vi "PCAN_WRITE.vi"(7 "path in":path, 8 "error in (no error)":errorcluster, 11 "TPCANMsg":T1={"ID"=0, "MSGTYPE"=128, "LEN"=0, "Data"=[]} {"ID" format="%x"; "MSGTYPE" items=["STATUS"=128, "EXTENDED"=2, "RTR"=1, "DATA MSG"=0]}) -> (0 "error out":errorcluster, 2 "path out":path, 3 "error":T2 items=["CAN_ERR_OK"=0, "CAN_ERR_XMTFULL"=1, "CAN_ERR_OVERRUN"=2, "CAN_ERR_BUSLIGHT"=4, "CAN_ERR_BUSHEAVY"=8, "CAN_ERR_BUSOFF"=16, "CAN_ERR_QRCVEMPTY"=32, "CAN_ERR_QOVERRUN"=64, "CAN_ERR_QXMTFULL"=128, "CAN_ERR_REGTEST"=256, "CAN_ERR_NOVXD"=512, "CAN_ERR_HWINUSE"=1024, "CAN_ERR_NETINUSE"=2048, "CAN_ERR_ILLHW"=5120, "CAN_ERR_ILLNET"=6144, "CAN_ERR_ILLCLINET"=7168, "CAN_ERR_RESOURCE"=8192, "CAN_ERR_ILLPARAMTYPE"=16384, "CAN_ERR_ILLPARAMVAL"=32768, "CAN_ERR_UNKNOWN"=65536])   [LabVIEW 2017]
doc: "///////////////////////////////////////////////////////////////////////////////\n// CAN_Write()\n// Schreibt eine Message \n// moegliche Fehler: NOVXD RESOURCE BUSOFF QXMTFULL\n//\n\nDWORD __stdcall CAN_Write( TPCANMsg* pMsgBuff);"
uses:
  PCAN_ERROR.ctl
  PCAN_USB.dll
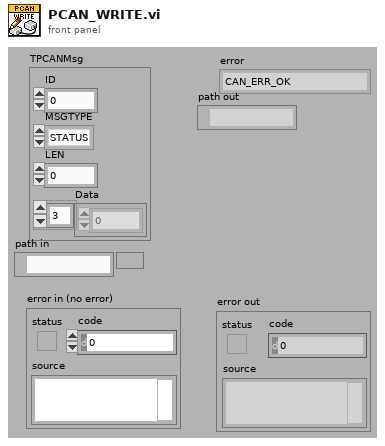
[diagram p1: front panel]
types:
  T1 = cluster{"ID":u32, "MSGTYPE":u8, "LEN":u8, "Data":u8[]}
  T2 = typedef "PCAN_ERROR.ctl" = i32
  T3 = enum16{"big-endian, network order", "native, host order", "little-endian"}
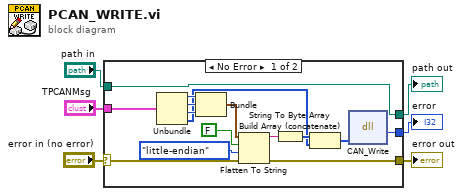
[diagram p0: block diagram]
diagram:
  n1 = case shown="No Error" "error in (no error)" {
    selector: "error in (no error)" -> [w9 w23]
    tunnel: [w21 _] -> w4
    tunnel: [w8 w23] -> w5
    tunnel: "TPCANMsg" -> [w20 _]
    tunnel: "path in" -> [w7 w22]
    tunnel: [w7 w22] -> w1
    frame No Error {
      n2 = Unbundle(w20) -> ("ID"=w19:u32, "MSGTYPE"=w18:u8, "LEN"=w17:u8, "Data"=w13:u8[])
      n3 = Bundle("ID"=w19, "MSGTYPE"=w18, "LEN"=w17) -> (w16:cluster{"ID":u32, "MSGTYPE":u8, "LEN":u8})  [unwired: 1 out]
      n4 = Flatten To String(anything=w16, prepend array or string size? (T)=FALSE, byte order (0:big-endian, network order)=T3."little-endian", error in (no error)=w9) -> (data string=w15:string, error out=w8:errorcluster)  [unwired: 1 out]
      n5 = String To Byte Array(string=w15) -> (unsigned byte array=w14:u8[])
      n6 = Build Array (concatenate)(w14, w13) -> (w12:u8[])
      n7 = dll-call lib="C:/Projects/Fuse_LW/Fuse25A_Labview/CANalystII/PCAN_USB.dll" fn="CAN_Write"("pMsgBuff"=w12) -> ("return type"=w21:i32)  [unwired: 4 in, 2 out]
    }
    frame Error {
    }
  }
  "error out" <- w5
  "error" <- w4
  "path out" <- w1
